vi "Start Async.vi"(8 "error in (no error)":errorcluster, 11 "gRPC service in":refnum<class "Manager.lvclass">) -> (0 "error out":errorcluster, 3 "gRPC service out":refnum<class "Manager.lvclass">)   [LabVIEW 2021, in "CIF_Manager_server.lvlib" / "Manager.lvclass"]
uses:
  Manager.lvclass
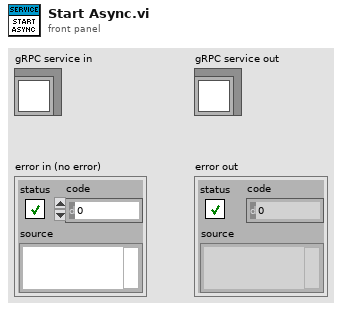
[diagram p1: front panel]
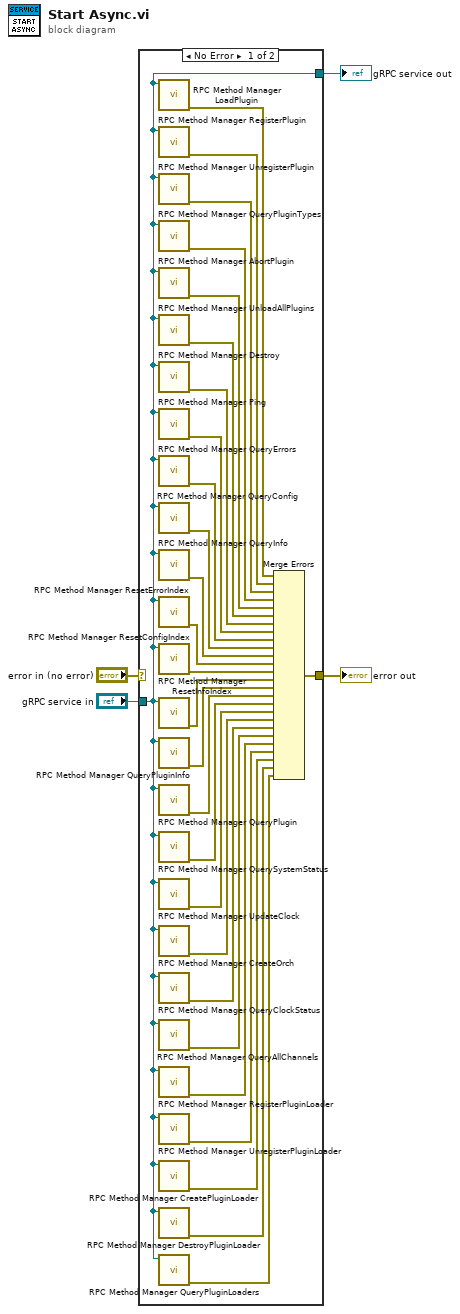
[diagram p0: block diagram]
diagram:
  n1 = case shown="No Error" "error in (no error)" {
    selector: "error in (no error)" -> [_ w34]
    tunnel: [w32 w34] -> w3
    tunnel: [w31 w33] -> w1
    tunnel: "gRPC service in" -> [w31 w33]
    frame No Error {
      n2 = call "RPC Method Manager LoadPlugin.vi"("gRPC service in"=w31) -> ("error out"=w30:errorcluster)  [unwired: 9 in, 1 out]
      n3 = call "RPC Method Manager RegisterPlugin.vi"("gRPC service in"=w31) -> ("error out"=w29:errorcluster)  [unwired: 9 in, 1 out]
      n4 = call "RPC Method Manager UnregisterPlugin.vi"("gRPC service in"=w31) -> ("error out"=w28:errorcluster)  [unwired: 9 in, 1 out]
      n5 = call "RPC Method Manager QueryPluginTypes.vi"("gRPC service in"=w31) -> ("error out"=w27:errorcluster)  [unwired: 9 in, 1 out]
      n6 = call "RPC Method Manager AbortPlugin.vi"("gRPC service in"=w31) -> ("error out"=w26:errorcluster)  [unwired: 9 in, 1 out]
      n7 = call "RPC Method Manager UnloadAllPlugins.vi"("gRPC service in"=w31) -> ("error out"=w25:errorcluster)  [unwired: 9 in, 1 out]
      n8 = call "RPC Method Manager Destroy.vi"("gRPC service in"=w31) -> ("error out"=w24:errorcluster)  [unwired: 9 in, 1 out]
      n9 = call "RPC Method Manager Ping.vi"("gRPC service in"=w31) -> ("error out"=w23:errorcluster)  [unwired: 9 in, 1 out]
      n10 = call "RPC Method Manager QueryErrors.vi"("gRPC service in"=w31) -> ("error out"=w22:errorcluster)  [unwired: 9 in, 1 out]
      n11 = call "RPC Method Manager QueryConfig.vi"("gRPC service in"=w31) -> ("error out"=w21:errorcluster)  [unwired: 9 in, 1 out]
      n12 = call "RPC Method Manager QueryInfo.vi"("gRPC service in"=w31) -> ("error out"=w20:errorcluster)  [unwired: 9 in, 1 out]
      n13 = call "RPC Method Manager ResetErrorIndex.vi"("gRPC service in"=w31) -> ("error out"=w19:errorcluster)  [unwired: 9 in, 1 out]
      n14 = call "RPC Method Manager ResetConfigIndex.vi"("gRPC service in"=w31) -> ("error out"=w18:errorcluster)  [unwired: 9 in, 1 out]
      n15 = call "RPC Method Manager ResetInfoIndex.vi"("gRPC service in"=w31) -> ("error out"=w17:errorcluster)  [unwired: 9 in, 1 out]
      n16 = call "RPC Method Manager QueryPluginInfo.vi"("gRPC service in"=w31) -> ("error out"=w16:errorcluster)  [unwired: 9 in, 1 out]
      n17 = call "RPC Method Manager QueryPlugin.vi"("gRPC service in"=w31) -> ("error out"=w15:errorcluster)  [unwired: 9 in, 1 out]
      n18 = call "RPC Method Manager QuerySystemStatus.vi"("gRPC service in"=w31) -> ("error out"=w14:errorcluster)  [unwired: 9 in, 1 out]
      n19 = call "RPC Method Manager UpdateClock.vi"("gRPC service in"=w31) -> ("error out"=w13:errorcluster)  [unwired: 9 in, 1 out]
      n20 = call "RPC Method Manager CreateOrch.vi"("gRPC service in"=w31) -> ("error out"=w12:errorcluster)  [unwired: 9 in, 1 out]
      n21 = call "RPC Method Manager QueryClockStatus.vi"("gRPC service in"=w31) -> ("error out"=w11:errorcluster)  [unwired: 9 in, 1 out]
      n22 = call "RPC Method Manager QueryAllChannels.vi"("gRPC service in"=w31) -> ("error out"=w10:errorcluster)  [unwired: 9 in, 1 out]
      n23 = call "RPC Method Manager RegisterPluginLoader.vi"("gRPC service in"=w31) -> ("error out"=w9:errorcluster)  [unwired: 9 in, 1 out]
      n24 = call "RPC Method Manager UnregisterPluginLoader.vi"("gRPC service in"=w31) -> ("error out"=w8:errorcluster)  [unwired: 9 in, 1 out]
      n25 = call "RPC Method Manager CreatePluginLoader.vi"("gRPC service in"=w31) -> ("error out"=w7:errorcluster)  [unwired: 9 in, 1 out]
      n26 = call "RPC Method Manager DestroyPluginLoader.vi"("gRPC service in"=w31) -> ("error out"=w6:errorcluster)  [unwired: 9 in, 1 out]
      n27 = call "RPC Method Manager QueryPluginLoaders.vi"("gRPC service in"=w31) -> ("error out"=w5:errorcluster)  [unwired: 9 in, 1 out]
      n28 = Merge Errors(w30, w29, w28, w27, w26, w25, w24, w23, w22, w21, w20, w19, w18, w17, w16, w15, w14, w13, w12, w11, w10, w9, w8, w7, w6, w5) -> (w32:errorcluster)
    }
    frame Error {
    }
  }
  "error out" <- w3
  "gRPC service out" <- w1
